vi "Write MultiBandConfig.vi"(8 "error in (no error)":errorcluster, 10 "MultiBandConfig":T1, 11 "MultiBandState in":refnum<class "MultiBandState.lvclass">) -> (0 "error out":errorcluster, 3 "MultiBandState out":refnum<class "MultiBandState.lvclass">)   [LabVIEW 2014, in "Functions.lvlib" / "MultiBandState.lvclass"]
uses:
  MultiBandState.lvclass
  TypeDefs/clMultiBandConfig.ctl
  TypeDefs/MultiBandConfig.ctl
  MultiBandState.lvclass/MultiBandState.ctl
panel:
  # "Band"
  # "Band"
  # "Band"
  # "Band"
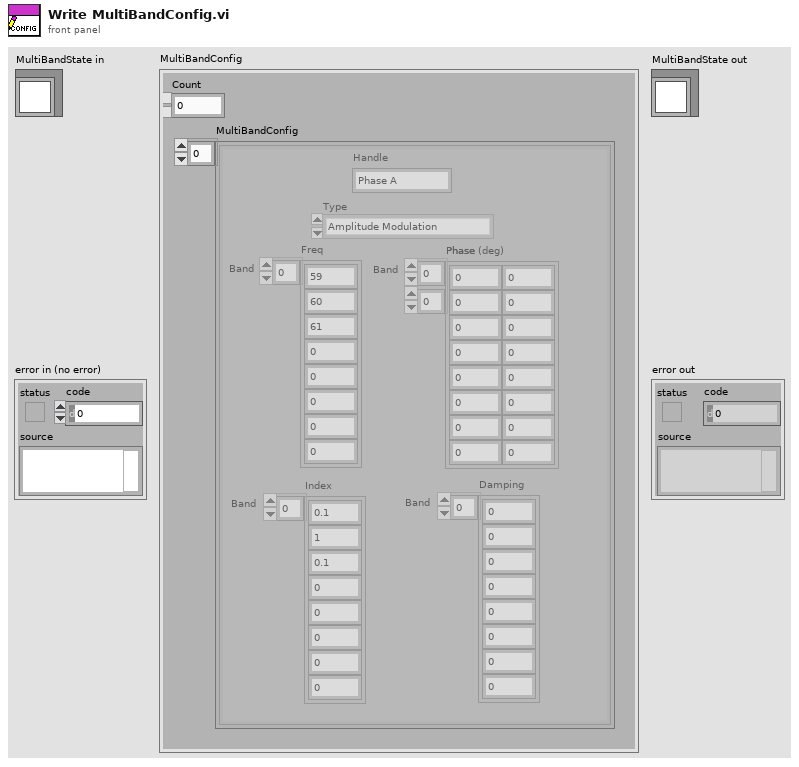
[diagram p1: front panel]
types:
  T1 = typedef "Functions.lvlib/MultiBandState.lvclass/clMultiBandConfig.ctl" = cluster{"Count":i32, "MultiBandConfig":T2[]}
  T2 = typedef "Functions.lvlib/MultiBandState.lvclass/MultiBandConfig.ctl" = cluster{"Handle":string, "Type":enum16{"Multiband", "Amplitude Modulation", "Phase Modulation", "Combined Modulation"}, "Freq":dbl[], "Index":dbl[], "Phase":dbl[][], "Damping":dbl[]}
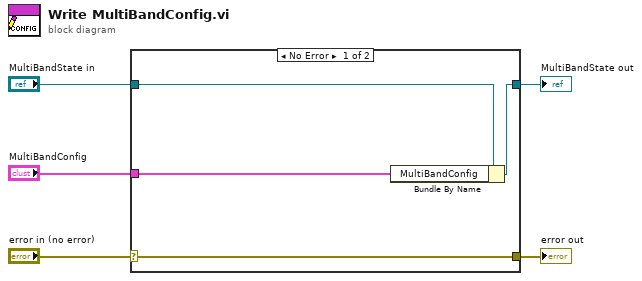
[diagram p0: block diagram]
diagram:
  n1 = case shown="No Error" "error in (no error)" {
    selector: "error in (no error)" -> [w9 w10]
    tunnel: [w9 w10] -> w4
    tunnel: [w7 w11] -> w2
    tunnel: "MultiBandState in" -> [w8 w11]
    tunnel: "MultiBandConfig" -> [w6 _]
    frame No Error {
      n2 = Bundle By Name(cluster=w8, "MultiBandConfig"=w6) -> (w7:refnum<class "MultiBandState.lvclass">)
    }
    frame Error {
    }
  }
  "error out" <- w4
  "MultiBandState out" <- w2
